vi "Tab Control - Change to TabName 24hr.vi"(1 "Label.Text":string, 3 "Status Tabl 3":refnum<vi>) -> ()   [LabVIEW 2014]
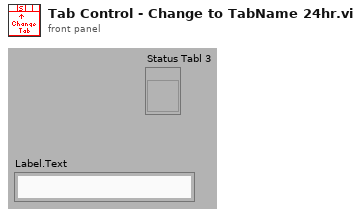
[diagram p1: front panel]
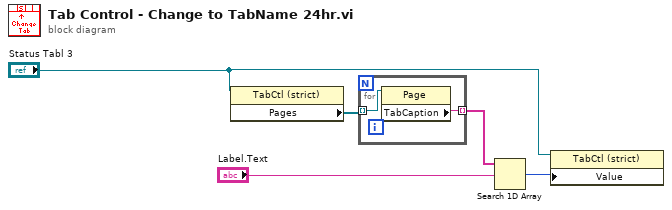
[diagram p0: block diagram]
diagram:
  n1 = property class="TabCtl (strict)"(reference="Status Tabl 3") -> ("Pages"=w5:refnum<vi>[])  [unwired: 1 in, 2 out]
  n2 = for {
    tunnel: w5 -> [w6] mode=indexing
    tunnel: [w7] -> w4 mode=indexing
    n3 = property class="Page"(reference=w6) -> ("TabCaption"=w7:string)  [unwired: 1 in, 2 out]
  }
  n4 = Search 1D Array(1D array=w4, element="Label.Text") -> (index of element=w2:i32)  [unwired: 1 in]
  n5 = property class="TabCtl (strict)"(reference="Status Tabl 3", "Value"=w2) -> ()  [unwired: 1 in, 2 out]
